vi "Write Waveform parameters.vi"(8 "error in (no error)":errorcluster, 10 "Waveform parameters":T1={"Sample rate"=6389760000.0, "Carrier frequency"=217000000.0, "Carrier amplitude"=30000.0, "Number of waves"=75.0, "Standard deviation"=0.1, "Add trigger wfrm"=TRUE} {"Carrier amplitude" format="%#_6p"; "Standard deviation" format="%#_6p"; "Number of waves" format="%#_6p"; "Carrier frequency" format="%#_6pHz"; "Sample rate" format="%#_6pHz"}, 11 "RFSoC Driver in":refnum<class "RFSoC Driver.lvclass">) -> (0 "error out":errorcluster, 3 "RFSoC Driver out":refnum<class "RFSoC Driver.lvclass">)   [LabVIEW 2019, in "RFSoC Driver.lvclass"]
uses:
  RFSoC Driver.lvclass
  Utilities/Waveform/Pulse Waveform Parameters.ctl
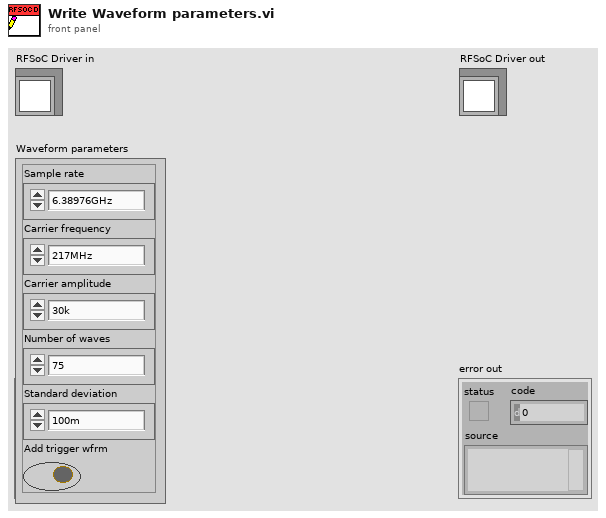
[diagram p1: front panel]
types:
  T1 = typedef "Pulse Waveform Parameters.ctl" = cluster{"Sample rate":dbl, "Carrier frequency":dbl, "Carrier amplitude":dbl, "Number of waves":dbl, "Standard deviation":dbl, "Add trigger wfrm":bool}
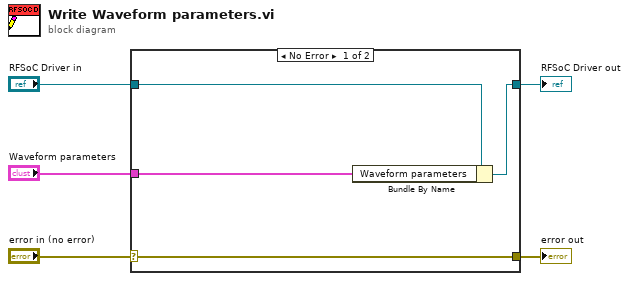
[diagram p0: block diagram]
diagram:
  n1 = case shown="No Error" "error in (no error)" {
    selector: "error in (no error)" -> [w9 w10]
    tunnel: [w9 w10] -> w4
    tunnel: [w7 w11] -> w2
    tunnel: "RFSoC Driver in" -> [w8 w11]
    tunnel: "Waveform parameters" -> [w6 _]
    frame No Error {
      n2 = Bundle By Name(cluster=w8, "Waveform parameters"=w6) -> (w7:refnum<class "RFSoC Driver.lvclass">)
    }
    frame Error {
    }
  }
  "error out" <- w4
  "RFSoC Driver out" <- w2
